vi "ReceiveNorification.vi"(8 "error in (no error)":errorcluster, 11 "GeneralDisplay in":refnum<class "SMS Notification.lvclass">) -> (0 "error out":errorcluster, 3 "GeneralDisplay out":refnum<class "SMS Notification.lvclass">)   [LabVIEW 2020, in "SMS Notification.lvclass"]
uses:
  SMS Notification.lvclass
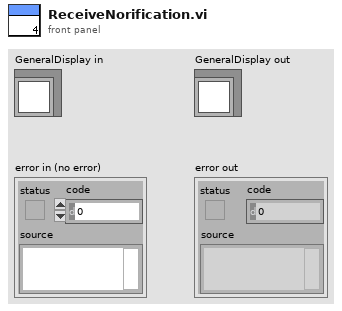
[diagram p1: front panel]
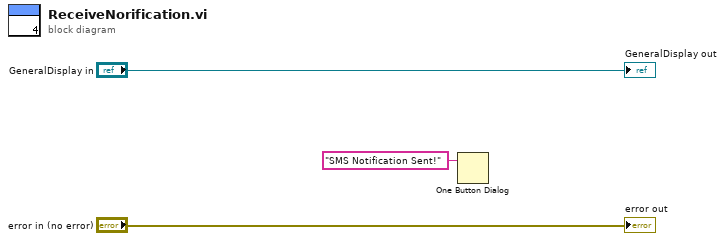
[diagram p0: block diagram]
diagram:
  n1 = One Button Dialog(message="SMS Notification Sent!") -> ()  [unwired: 1 in, 1 out]
  "error out" <- "error in (no error)"
  "GeneralDisplay out" <- "GeneralDisplay in"
